vi "DefenderStop.vi"(6 "Defensores":u32[](array[numeric]), 7 "total":i32, 9 "Field Size in":T1, 10 "balls":T4[](array[typedef]), 11 "Our Robot in":T2) -> (2 "Robot out":T2)   [LabVIEW 2016]
uses:
  Core/AI Robot.ctl
  Functions Enum.ctl
  Core/AI Ball.ctl
  Core/Field Size.ctl
panel:
  in  "Radius":i32=40
  in  "Stretch":i32=60
  in  "D max":dbl=500.0
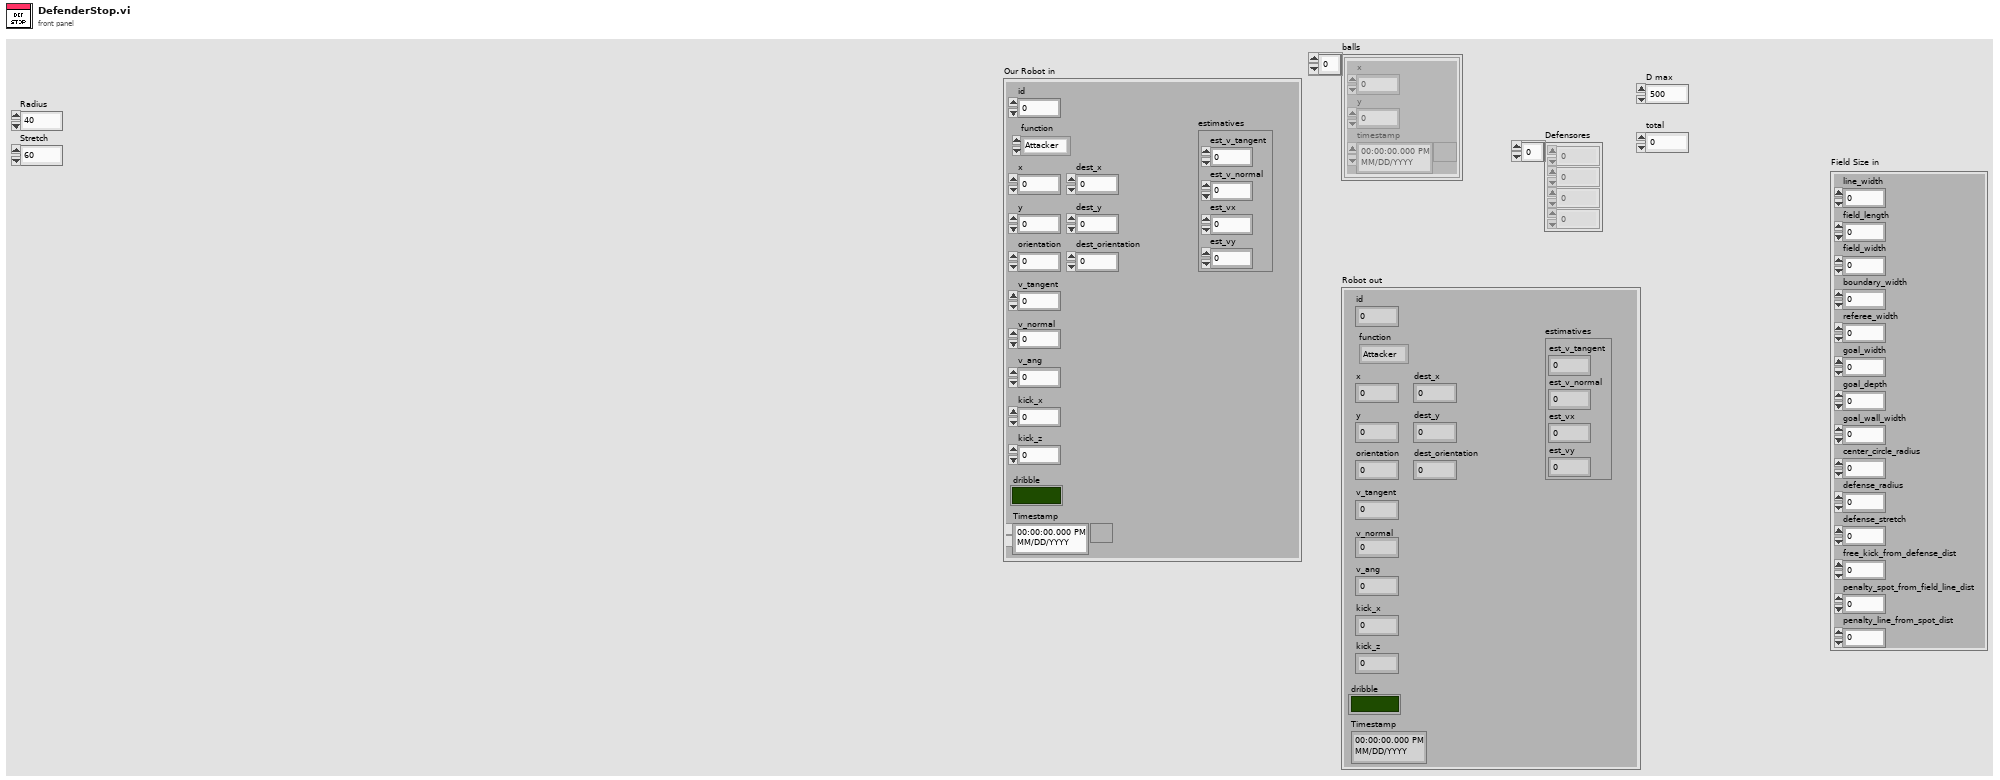
[diagram p1: front panel]
types:
  T1 = typedef "Field Size.ctl" = cluster{"line_width":u32, "field_length":u32, "field_width":u32, "boundary_width":u32, "referee_width":u32, "goal_width":u32, "goal_depth":u32, "goal_wall_width":u32, "center_circle_radius":u32, "defense_radius":u32, "defense_stretch":u32, "free_kick_from_defense_dist":u32, "penalty_spot_from_field_line_dist":u32, "penalty_line_from_spot_dist":u32}
  T2 = typedef "AI Robot.ctl" = cluster{"id":u32, "function":T3, "x":dbl, "y":dbl, "orientation":dbl, "v_tangent":dbl, "v_normal":dbl, "v_ang":dbl, "kick_x":dbl, "kick_z":dbl, "dribble":bool, "Timestamp":timestamp, "dest_x":dbl, "dest_y":dbl, "dest_orientation":dbl, "estimatives":cluster{"est_v_tangent":dbl, "est_v_normal":dbl, "est_vx":dbl, "est_vy":dbl}}
  T3 = typedef "Functions Enum.ctl" = enum16{"Attacker", "Goalie", "Defender", "Striker", "Goto 0", "Dummy", "ZigZag"}
  T4 = typedef "AI Ball.ctl" = cluster{"x":dbl, "y":dbl, "timestamp":timestamp}
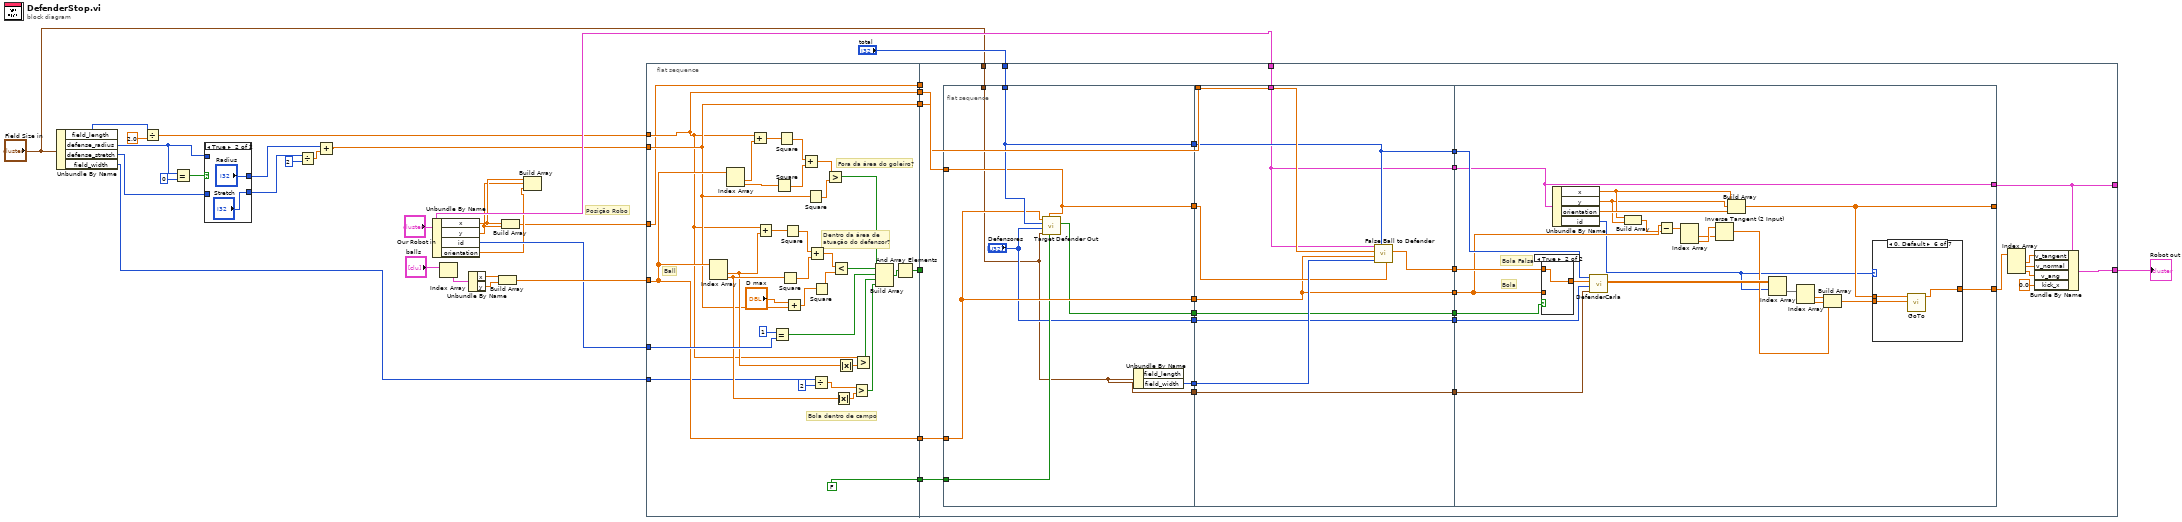
[diagram p0: block diagram]
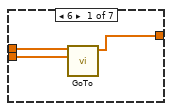
[diagram p3: hidden frame]
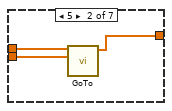
[diagram p4: hidden frame]
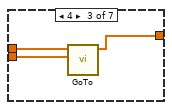
[diagram p5: hidden frame]
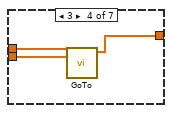
[diagram p6: hidden frame]
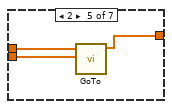
[diagram p7: hidden frame]
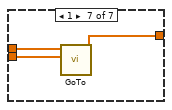
[diagram p8: hidden frame]
diagram:
  # "Posição Robo"
  n1 = Unbundle By Name("Field Size in") -> ("field_length"=w11:u32, "defense_radius"=w9:u32, "defense_stretch"=w8:u32, "field_width"=w1:u32)
  n2 = Divide(x=w11, y=2.0) -> (x/y=w2:dbl)
  n3 = Equal?(x=w9, y=u32 0) -> (x = y?=w7:bool)
  n4 = case shown="True" w7 {
    tunnel: [w35 "Radius"] -> w6
    tunnel: w9 -> [w35 _]
    tunnel: w8 -> [w34 _]
    tunnel: [w34 "Stretch"] -> w5
    frame False {
    }
    frame True {
    }
  }
  n5 = Divide(x=w5, y=u32 2) -> (x/y=w14:dbl)
  n6 = Add(x=w6, y=w14) -> (x+y=w3:dbl)
  n7 = Unbundle By Name("Our Robot in") -> ("x"=w26:dbl, "y"=w25:dbl, "id"=w28:u32, "orientation"=w24:dbl)
  n8 = Index Array(array="balls") -> (element=w32:T4)  [unwired: 1 in]
  n9 = Unbundle By Name(w32) -> ("x"=w31:dbl, "y"=w30:dbl)
  n10 = Build Array(w31, w30) -> (w29:dbl[])
  n11 = Build Array(w26, w25) -> (w23:dbl[])
  n12 = Build Array(w26, w25, w24) -> ()  [unwired: 1 out]
  n13 = flat-sequence {
    tunnel: w3 -> [w40]
    tunnel: w2 -> [w39]
    tunnel: w29 -> [w56]
    tunnel: w23 -> [w38]
    tunnel: [w56] -> w22
    tunnel: [w63] -> w21
    tunnel: w28 -> [w62]
    tunnel: w1 -> [w47]
    tunnel: [FALSE ("Target Fora")] -> w20
    tunnel: [w39] -> w19
    tunnel: [w40] -> w18
    tunnel: [w38] -> w17
    tunnel: "total" -> [w100]
    tunnel: [w99] -> w15
    tunnel: w22 -> [w98]
    tunnel: w21 -> [_]
    tunnel: w20 -> [w97]
    tunnel: w19 -> [w95]
    tunnel: "Field Size in" -> [w96]
    tunnel: "Our Robot in" -> [w94]
    tunnel: w18 -> [w93]
    tunnel: [w92] -> _
    tunnel: w17 -> [_]
    frame #0 {
      # "Bola dentro de campo"
      # "Dentro da área de \natuação do defensor?"
      # "Fora da área do goleiro?"
      # "Ball"
      n14 = Index Array(array=w56) -> (element #1=w44:dbl, element #2=w48:dbl)  [unwired: 2 in]
      n15 = Index Array(array=w56) -> (element #1=w64:dbl, element #2=w66:dbl)  [unwired: 2 in]
      n16 = Add(x=w39, y=w64) -> (x+y=w65:dbl)
      n17 = Add(x=w39, y=w44) -> (x+y=w57:dbl)
      n18 = Equal?(x=u32 1, y=w62) -> (x = y?=w60:bool)
      n19 = Square(x=w66) -> (x^2=w68:dbl)
      n20 = Square(x=w65) -> (x^2=w67:dbl)
      n21 = Square(x=w48) -> (x^2=w59:dbl)
      n22 = Square(x=w57) -> (x^2=w58:dbl)
      n23 = Add(x="D max", y=w40) -> (x+y=w42:dbl)
      n24 = Add(x=w67, y=w68) -> (x+y=w69:dbl)
      n25 = Square(x=w40) -> (x^2=w70:dbl)
      n26 = Add(x=w58, y=w59) -> (x+y=w53:dbl)
      n27 = Divide(x=w47, y=u32 2) -> (x/y=w50:dbl)
      n28 = Square(x=w42) -> (x^2=w55:dbl)
      n29 = Greater?(x=w69, y=w70) -> (0:w71:bool)
      n30 = Less?(x=w53, y=w55) -> (x < y?=w54:bool)
      n31 = Absolute Value(x=w48) -> (abs(x)=w49:dbl)
      n32 = Absolute Value(x=w44) -> (abs(x)=w52:dbl)
      n33 = Greater?(x=w50, y=w49) -> (0:w45:bool)
      n34 = Greater?(x=w39, y=w52) -> (0:w51:bool)
      n35 = Build Array(w71, w54, w60, w51, w45) -> (w72:bool[])
      n36 = And Array Elements(Boolean array=w72) -> (logical AND=w63:bool)
    }
    frame #1 {
      n37 = flat-sequence {
        tunnel: w100 -> [w107]
        tunnel: [w108] -> w91
        tunnel: w98 -> [w106]
        tunnel: [w107] -> w90
        tunnel: w97 -> [w104]
        tunnel: w95 -> [w105]
        tunnel: w96 -> [w101]
        tunnel: [w106] -> w89
        tunnel: [w105] -> w88
        tunnel: [w103] -> w87
        tunnel: ["Defensores"] -> w86
        tunnel: [w101] -> w85
        tunnel: w91 -> [w118]
        tunnel: w90 -> [w112]
        tunnel: w94 -> [w109]
        tunnel: w93 -> [w117]
        tunnel: w89 -> [w114]
        tunnel: w88 -> [w116]
        tunnel: [w115] -> w84
        tunnel: [w114] -> w83
        tunnel: [w113] -> w82
        tunnel: w87 -> [w113]
        tunnel: [w112] -> w81
        tunnel: [w111] -> w80
        tunnel: w86 -> [w111]
        tunnel: [w110] -> w79
        tunnel: w85 -> [w110]
        tunnel: [w109] -> w78
        tunnel: [w135] -> w73
        tunnel: [w128] -> w92
        tunnel: w84 -> [w133]
        tunnel: w83 -> [w129]
        tunnel: w82 -> [w132]
        tunnel: w81 -> [w131]
        tunnel: w80 -> [w130]
        tunnel: w79 -> [w127]
        tunnel: w78 -> [w128]
        tunnel: [w121] -> _
        frame #0 {
          n38 = call "Target Defender Out.vi"("Target Fora in"=w104, "Campo/2"=w105, "Field Size in"=w101, "Defensores"="Defensores", "total"=w107, "Ball"=w106) -> ("Target Fora out"=w103:bool)  [unwired: 5 in]
          n39 = Unbundle By Name(w101) -> ("field_width"=w108:u32)  [unwired: 1 out]
        }
        frame #1 {
          n40 = call "False Ball to Defender.vi"("Campo/2"=w116, "field_width"=w118, "total"=w112, "Bola"=w114, "raio da área \ndo goleiro"=w117, "Our Robot in"=w109) -> ("Bola Falsa"=w115:dbl[])  [unwired: 5 in]
        }
        frame #2 {
          # "Bola"
          # "Bola Falsa"
          n41 = case shown="True" w132 {
            tunnel: [w164 w165] -> w142
            tunnel: w133 -> [_ w165]
            tunnel: w129 -> [w164 _]
            frame False {
            }
            frame True {
            }
          }
          n42 = Unbundle By Name(w128) -> ("x"=w140:dbl, "y"=w139:dbl, "orientation"=w141:dbl, "id"=w119:u32)
          n43 = call "DefenderCarla.vi"("Field Size in"=w127, "Defensores"=w130, "Ball"=w142, "total"=w131) -> ("Posição dos Defensores"=w125:dbl[][])  [unwired: 6 in]
          n44 = Build Array(w140, w139) -> (w126:dbl[])
          n45 = Subtract(x=w129, y=w126) -> (x-y=w138:dbl[])
          n46 = Index Array(array=w138) -> (element #1=w136:dbl, element #2=w137:dbl)  [unwired: 2 in]
          n47 = Inverse Tangent (2 Input)(1:w136, 2:w137) -> (0:w120:dbl)
          n48 = Build Array(w140, w139, w141) -> (w121:dbl[])
          n49 = Index Array(array=w125, index (row)=w119) -> (element=w124:dbl[])  [unwired: 1 in]
          n50 = Index Array(array=w124) -> (element #1=w123:dbl, element #2=w122:dbl)  [unwired: 2 in]
          n51 = Build Array(w123, w122, w120) -> (w134:dbl[])
          n52 = case shown="0, Default" w119 {
            tunnel: [w143 w146 w149 w152 w155 w158 w163] -> w135
            tunnel: w134 -> [w144 w148 w150 w153 w156 w159 w162]
            tunnel: w121 -> [w145 w147 w151 w154 w157 w160 w161]
            frame 6 {
              n53 = call "GoTo.vi"("Target"=w144, "Position"=w145) -> ("Output\nVelocity"=w143:dbl[])  [unwired: 8 in, 1 out]
            }
            frame 5 {
              n54 = call "GoTo.vi"("Target"=w148, "Position"=w147) -> ("Output\nVelocity"=w146:dbl[])  [unwired: 8 in, 1 out]
            }
            frame 4 {
              n55 = call "GoTo.vi"("Target"=w150, "Position"=w151) -> ("Output\nVelocity"=w149:dbl[])  [unwired: 8 in, 1 out]
            }
            frame 3 {
              n56 = call "GoTo.vi"("Target"=w153, "Position"=w154) -> ("Output\nVelocity"=w152:dbl[])  [unwired: 8 in, 1 out]
            }
            frame 2 {
              n57 = call "GoTo.vi"("Target"=w156, "Position"=w157) -> ("Output\nVelocity"=w155:dbl[])  [unwired: 8 in, 1 out]
            }
            frame 0, Default {
              n58 = call "GoTo.vi"("Target"=w159, "Position"=w160) -> ("Output\nVelocity"=w158:dbl[])  [unwired: 8 in, 1 out]
            }
            frame 1 {
              n59 = call "GoTo.vi"("Target"=w162, "Position"=w161) -> ("Output\nVelocity"=w163:dbl[])  [unwired: 8 in, 1 out]
            }
          }
        }
      }
      n60 = Index Array(array=w73) -> (element #1=w76:dbl, element #2=w75:dbl, element #3=w74:dbl)  [unwired: 3 in]
      n61 = Bundle By Name(cluster=w92, "v_tangent"=w76, "v_normal"=w75, "v_ang"=w74, "kick_x"=0.0) -> (w99:T2)
    }
  }
  "Robot out" <- w15
